vi "AAA Table Function Catalog.vi"   [LabVIEW 2010]
panel:
  # "Table Function\nCatalog"
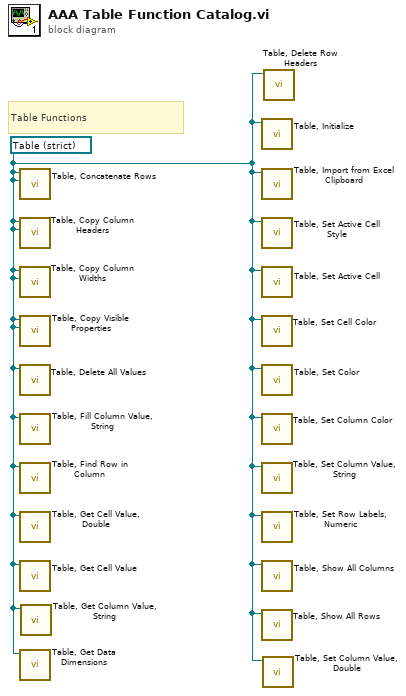
[diagram p0: block diagram]
diagram:
  w1 = refnum<vi> refnum ("Tbl Refnum Src")
  # "Table Functions"
  n1 = call "Table, Concatenate Rows.vi"("Tbl Refnum Dst"=w1, "Tbl Refnum Src"=w1) -> ()  [unwired: 3 in, 3 out]
  n2 = call "Table, Copy Column Headers.vi"("Tbl Refnum Dst"=w1, "Tbl Refnum Src"=w1) -> ()  [unwired: 3 in, 3 out]
  n3 = call "Table, Copy Column Widths.vi"("Tbl Refnum Dst"=w1, "Tbl Refnum Src"=w1) -> ()  [unwired: 3 in, 3 out]
  n4 = call "Table, Copy Visible Properties.vi"("Tbl Refnum Dst"=w1, "Tbl Refnum Src"=w1) -> ()  [unwired: 3 in, 3 out]
  n5 = call "Table, Delete All Values.vi"("Tbl Refnum"=w1) -> ()  [unwired: 9 in, 2 out]
  n6 = call "Table, Fill Column Value, String.vi"("Tbl Refnum"=w1) -> ()  [unwired: 9 in, 2 out]
  n7 = call "Table, Find Row in Column.vi"("Tbl Refnum"=w1) -> ()  [unwired: 7 in, 4 out]
  n8 = call "Table, Get Cell Value, Double.vi"("Tbl Refnum"=w1) -> ()  [unwired: 8 in, 3 out]
  n9 = call "Table, Get Cell Value.vi"("Tbl Refnum"=w1) -> ()  [unwired: 8 in, 3 out]
  n10 = call "Table, Get Data Dimensions.vi"("Tbl Refnum"=w1) -> ()  [unwired: 7 in, 4 out]
  n11 = call "Table, Get Column Value, String.vi"("Tbl Refnum"=w1) -> ()  [unwired: 7 in, 3 out]
  n12 = call "Table, Initialize.vi"("Tbl Refnum"=w1) -> ()  [unwired: 9 in, 2 out]
  n13 = call "Table, Import from Excel Clipboard.vi"("Tbl Refnum"=w1) -> ()  [unwired: 9 in, 2 out]
  n14 = call "Table, Set Active Cell Style.vi"("Tbl Refnum"=w1) -> ()  [unwired: 7 in, 2 out]
  n15 = call "Table, Set Active Cell.vi"("Tbl Refnum"=w1) -> ()  [unwired: 7 in, 2 out]
  n16 = call "Table, Set Cell Color.vi"("Tbl Refnum"=w1) -> ()  [unwired: 8 in, 2 out]
  n17 = call "Table, Set Color.vi"("Tbl Refnum"=w1) -> ()  [unwired: 8 in, 2 out]
  n18 = call "Table, Set Column Color.vi"("Tbl Refnum"=w1) -> ()  [unwired: 8 in, 2 out]
  n19 = call "Table, Set Column Value, String.vi"("Tbl Refnum"=w1) -> ()  [unwired: 8 in, 3 out]
  n20 = call "Table, Set Row Labels, Numeric.vi"("Tbl Refnum"=w1) -> ()  [unwired: 9 in, 2 out]
  n21 = call "Table, Show All Columns.vi"("Tbl Refnum"=w1) -> ()  [unwired: 9 in, 2 out]
  n22 = call "Table, Show All Rows.vi"("Tbl Refnum"=w1) -> ()  [unwired: 9 in, 2 out]
  n23 = call "Table, Set Column Value, Double.vi"("Tbl Refnum"=w1) -> ()  [unwired: 8 in, 3 out]
  n24 = call "Table, Delete Row Headers.vi"("Tbl Refnum"=w1) -> ()  [unwired: 9 in, 2 out]
